vi "Untitled 1.vi"() -> ()   [LabVIEW 2021]
uses:
  Lab 3 Template/State.ctl
panel:
  in  "stop":bool
  out "Intensity Chart":dbl[][](graph)
  out "Thermometer":dbl(slide) scale=0.0..100.0
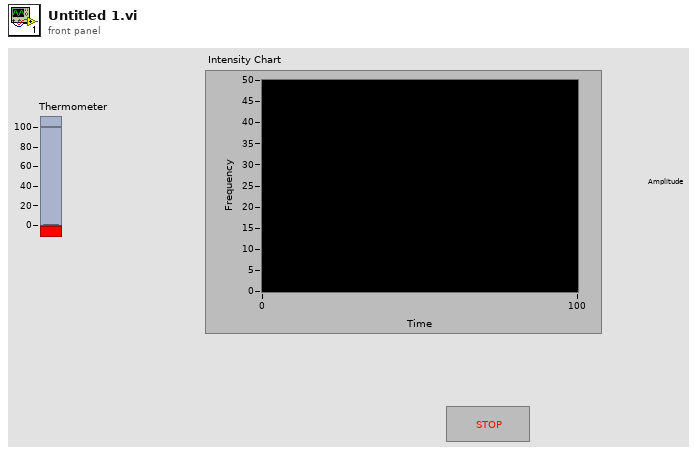
[diagram p1: front panel]
types:
  T1 = typedef "State.ctl" = enum16{"Reset", "Initialize", "Wait", "Shutdown"}
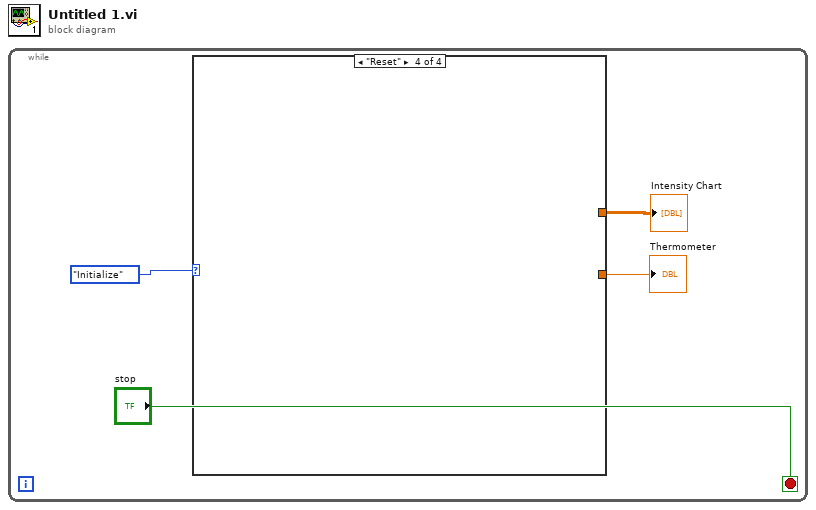
[diagram p0: block diagram]
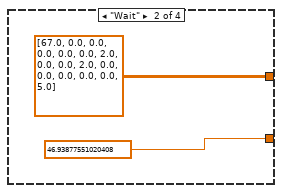
[diagram p3: hidden frame]
diagram:
  n1 = while {
    stop <- "stop" stop-if-true
    n2 = case shown="\"Reset\"" State."Initialize" {
      tunnel: [_ dbl[][] [[67.0, 0.0, 0.0, 0.0], [0.0, 0.0, 2.0, 0.0], [0.0, 2.0, 0.0, 0.0], [0.0, 0.0, 0.0, 5.0]] ("Intensity Chart") _ _] -> w3
      tunnel: [_ 46.93877551020408 ("Thermometer") _ _] -> w2
      frame "Initialize", Default {
      }
      frame "Wait" {
      }
      frame "Shutdown" {
      }
      frame "Reset" {
      }
    }
    "Intensity Chart" <- w3
    "Thermometer" <- w2
  }
